vi "IRH1-2M_Heuristic.vi"(10 "Scheduler":T1(ring), 11 "Proocessing Times":u16[][](array[numeric])=[[1, 69, 192, 47, 292, 28, 166, 205], [146, 96, 177, 62, 37, 145, 3, 34], [99, 182, 133, 113, 9, 239, 27, 198], [159, 182, 132, 158, 183, 38, 142, 6], [92, 63, 114, 144, 180, 199, 136, 72], [119, 31, 9, 163, 139, 158, 350, 31], [46, 30, 59, 290, 156, 90, 175, 154], [338, 347, 184, 23, 4, 103, 1, 0]]) -> (3 "IRH1 Schedule":u16[](array[numeric]))   [LabVIEW 2013]
uses:
  Classes/GanntChart.lvclass
panel:
  in  "Proocessing Times (8x8)":u16[][](array[numeric])=[[1, 69, 192, 47, 292, 28, 166, 205], [146, 96, 177, 62, 37, 145, 3, 334], [99, 182, 133, 113, 9, 239, 27, 198], [159, 182, 132, 158, 183, 38, 142, 6], [92, 63, 114, 144, 180, 199, 136, 72], [119, 31, 9, 163, 139, 158, 350, 31], [46, 30, 59, 290, 156, 90, 175, 154], [338, 347, 184, 23, 4, 103, 1, 0]]
  out "Machine Completion Times":u16[](array[numeric])
  out "Completion Times":u16[][](array[numeric])
  out "Job Completion Times":i32[](array[numeric])
  out "String":string
  out "LPT Array":i32[](array[numeric])
  out "Makespan":i32
  # "1, 69, 192, 47, 292, 28, 166, 205], \n[146, 96, 177, 62, 37, 145, 3, 334], \n[99, 182, 133, 113, 9, 239, 27, 198], \n[159, 182, 132, 158, 183, 38, 142, 6], \n[92, 63, 114, 144, 180, 199, 136, 72], \n[119, 31, 9, 163, 139, 158, 350, 31], \n[46, 30, 59, 290, 156, 90, 175, 154], \n[338, 347, 184, 23, 4, 103, 1, 0]]"
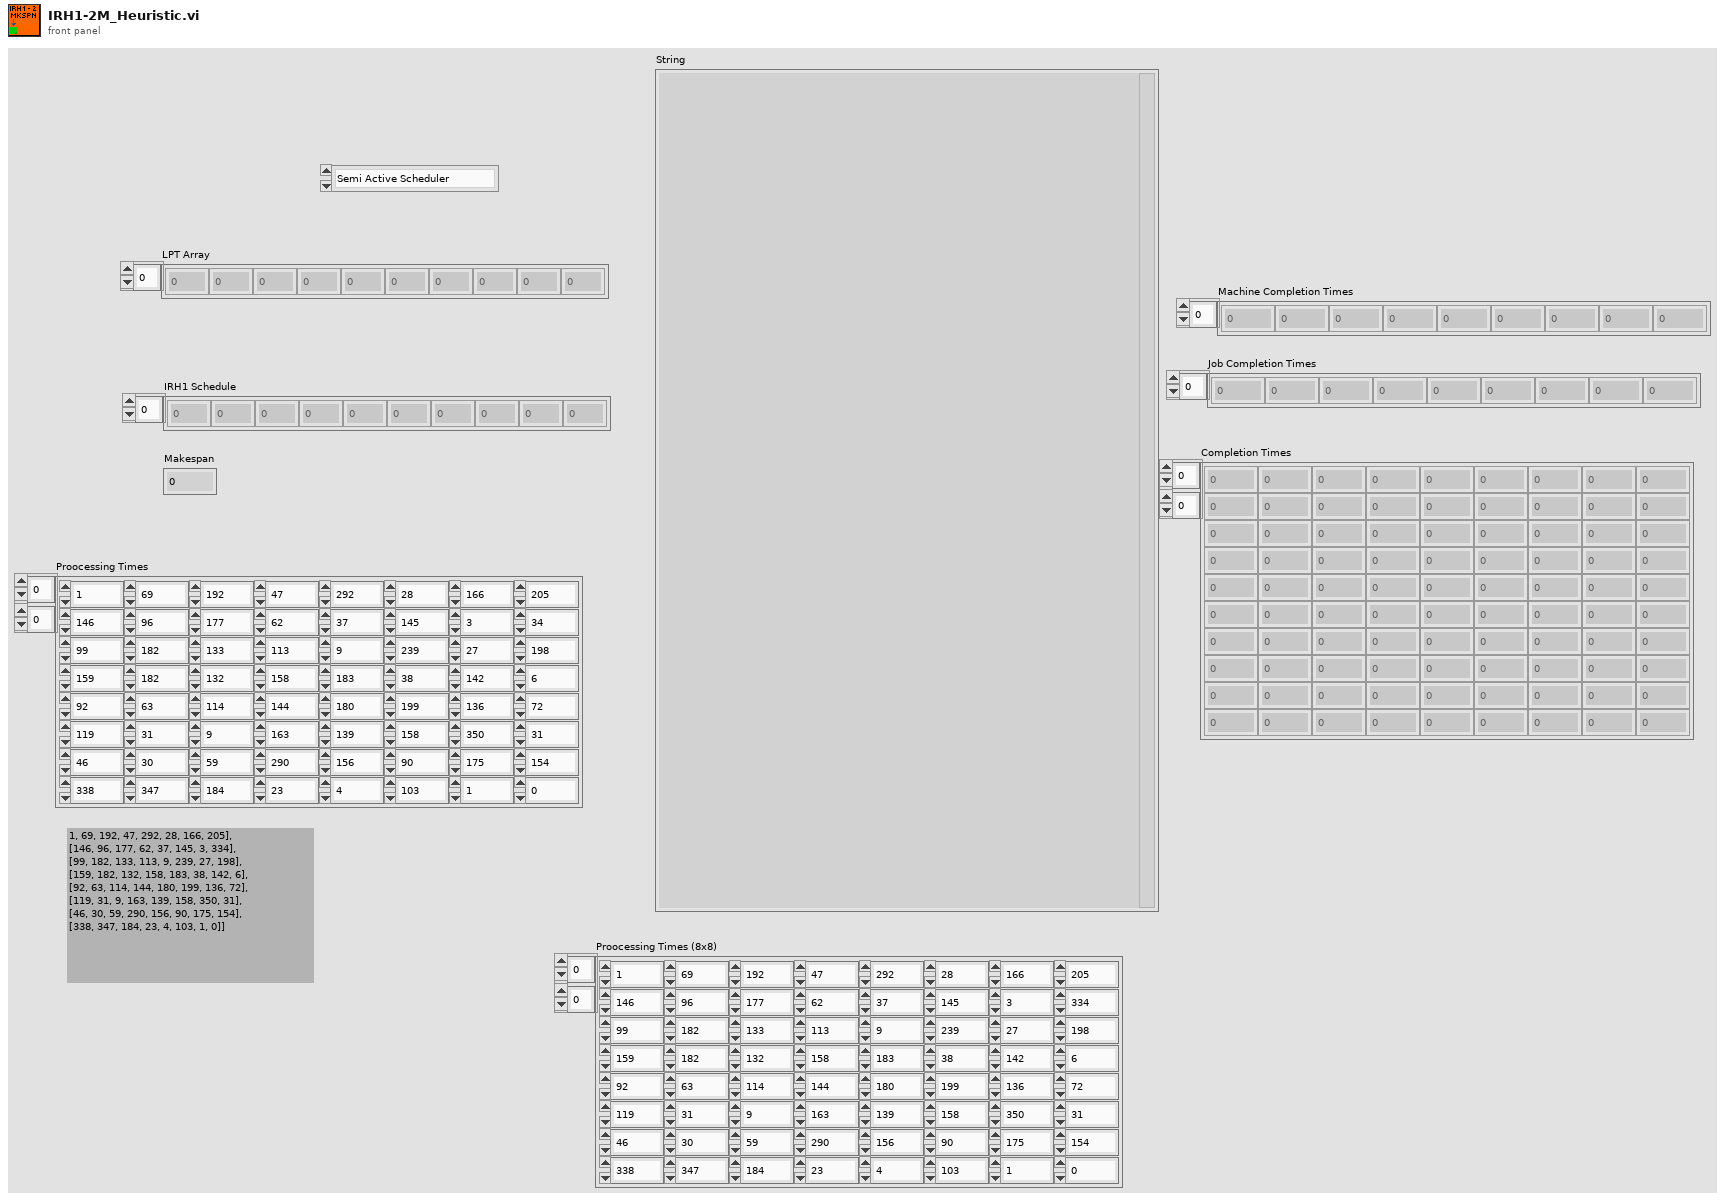
[diagram p1: front panel]
types:
  T1 = enum16{"Semi Active Scheduler", "Non Delay Scheduler"}
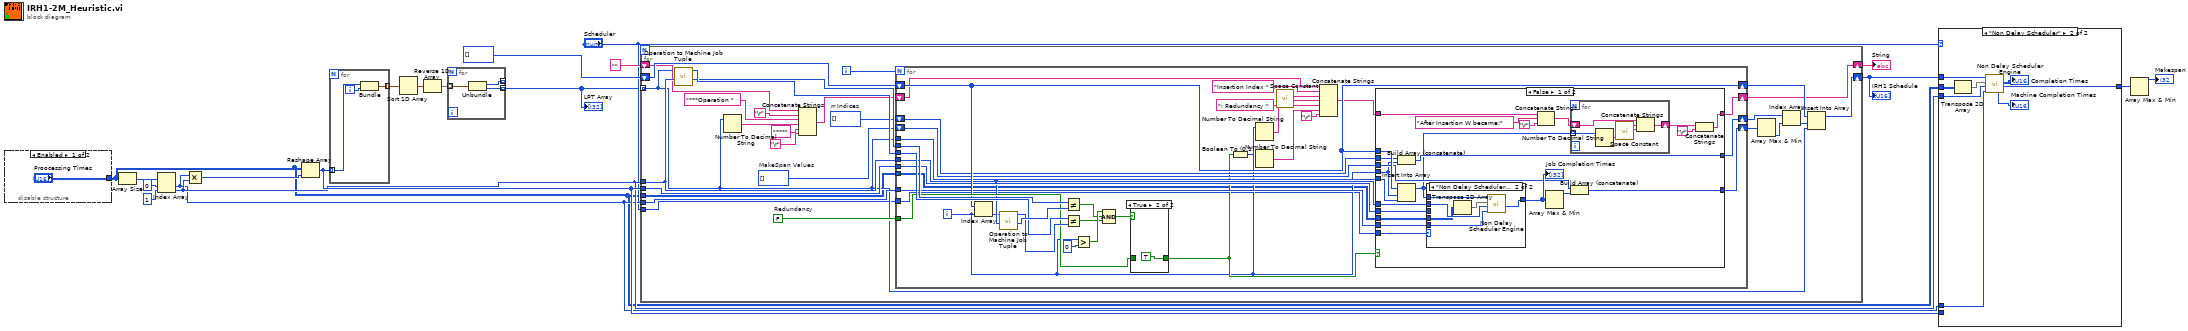
[diagram p0: block diagram]
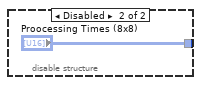
[diagram p2: hidden frame]
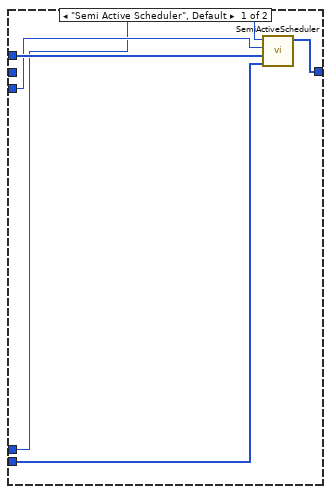
[diagram p3: hidden frame]
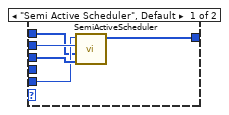
[diagram p4: hidden frame]
diagram:
  n1 = disable-structure shown="Enabled" {
    disable-tunnel: ["Proocessing Times" "Proocessing Times (8x8)"] -> w1
    frame Enabled {
    }
    frame Disabled {
    }
  }
  n2 = Array Size(array=w1) -> (size(s)=w18:i32[])
  n3 = Index Array(array=w18, index #1=0 ("index"), index #2=1 ("index")) -> (element #1=w8:i32, element #2=w9:i32)
  n4 = Multiply(x=w8, y=w9) -> (x*y=w13:i32)
  n5 = Reshape Array(w1, w13) -> (w10:u16[])
  n6 = for {
    tunnel: w10 -> [w24] mode=indexing
    tunnel: [w22] -> w15 mode=indexing
    i -> [w23]
    n7 = Bundle(w24, w23) -> (w22:cluster{u16, i32})  [unwired: 1 in]
  }
  n8 = Sort 1D Array(array=w15) -> (sorted array=w19:cluster{u16, i32}[])
  n9 = Reverse 1D Array(array=w19) -> (reversed array=w14:cluster{u16, i32}[])
  n10 = for {
    tunnel: w14 -> [w27] mode=indexing
    tunnel: [w26] -> _ mode=indexing
    tunnel: [w25] -> w2 mode=indexing
    n11 = Unbundle(w27) -> (w26:u16, w25:i32)
  }
  "LPT Array" <- w2
  n12 = for {
    tunnel: w2 -> [w36] mode=indexing
    tunnel: w9 -> [w48]
    shift-right: [w40] -> w11
    shift-left: u16[] [] -> [w52]
    tunnel: w10 -> [w41]
    tunnel: w8 -> [w47]
    shift-right: [w38] -> w4
    shift-left: "" -> [w37]
    tunnel: w1 -> [w29]
    tunnel: "Scheduler" -> [w28]
    i -> [w54]
    w45 = i32[] []  # MakeSpan Values
    w46 = i32[] []  # rr Indices
    w53 = FALSE  # Redundancy
    n13 = call "Operation to Machine Job Tuple.vi"("Number of Machines"=w48, "Operation Number"=w36) -> ("Job No"=w49:i32, "Machine No"=w50:i32)  [unwired: 8 in]
    n14 = Number To Decimal String(number=w36) -> (decimal integer string=w34:string)  [unwired: 1 in]
    n15 = Concatenate Strings(w37, "\r", "***Operation " ("string"), w34, "***" ("string"), "\r") -> (w33:string)
    n16 = for {
      N: w54 -> [_]
      shift-right: [w79] -> w51
      shift-left: w52 -> [w79]
      tunnel: w50 -> [w83]
      tunnel: w49 -> [w86]
      tunnel: w48 -> [w76]
      tunnel: w53 -> [w80]
      tunnel: w36 -> [w78]
      tunnel: w41 -> [w77]
      tunnel: w47 -> [w75]
      shift-right: [w73] -> w44
      shift-left: w46 -> [w74]
      shift-right: [w71] -> w39
      shift-left: w45 -> [w72]
      shift-right: [w69] -> w38
      shift-left: w33 -> [w63]
      tunnel: w29 -> [w56]
      tunnel: w28 -> [w55]
      i -> [w60]
      n17 = Index Array(array=w79, index=w60) -> (element=w68:u16)
      n18 = call "Operation to Machine Job Tuple.vi"("Number of Machines"=w76, "Operation Number"=w68) -> ("Job No"=w85:i32, "Machine No"=w82:i32)  [unwired: 8 in]
      n19 = Not Equal?(x=w86, y=w85) -> (x != y?=w84:bool)
      n20 = Not Equal?(x=w83, y=w82) -> (x != y?=w70:bool)
      n21 = Greater?(x=w60, y=0) -> (0:w87:bool)
      n22 = Compound Arithmetic op=AND(w87, w84, w70) -> (w81:bool)
      n23 = case shown="True" w81 {
        tunnel: w80 -> [w130 _]
        tunnel: [w130 TRUE ("Redundancy")] -> w61
        frame False {
        }
        frame True {
        }
      }
      n24 = Boolean To (0,1)(Boolean=w61) -> (0, 1=w59:i16)
      n25 = Number To Decimal String(number=w60) -> (decimal integer string=w65:string)  [unwired: 1 in]
      n26 = Number To Decimal String(number=w59) -> (decimal integer string=w58:string)  [unwired: 1 in]
      n27 = call <vilib>:"Space Constant.vi"() -> ("String"=w66:string)
      n28 = Concatenate Strings(w63, "Insertion Index " ("string"), w65, w66, "; Redundancy " ("string"), w58, "\r") -> (w62:string)
      n29 = case shown="False" w61 {
        tunnel: w79 -> [w110 _]
        tunnel: w78 -> [w109 _]
        tunnel: w77 -> [w108 _]
        tunnel: w76 -> [w107 _]
        tunnel: w75 -> [w106 _]
        tunnel: w74 -> [w105 w129]
        tunnel: w60 -> [w97 _]
        tunnel: [w104 w129] -> w73
        tunnel: w72 -> [w102 w128]
        tunnel: [w100 w128] -> w71
        tunnel: [w98 w127] -> w69
        tunnel: w62 -> [w96 w127]
        tunnel: w56 -> [w89 _]
        tunnel: w55 -> [w90 _]
        frame False {
          n30 = Build Array (concatenate)(w105, w97) -> (w104:i32[])
          n31 = Insert Into Array(array=w110, index=w97, new element=w109) -> (w99:u16[])
          n32 = case shown="\"Non Delay Scheduler\"" w90 {
            tunnel: w108 -> [w115 _]
            tunnel: w107 -> [w114 w120]
            tunnel: w106 -> [w113 w119]
            tunnel: [w112 w118] -> w103
            tunnel: w99 -> [w111 w121]
            tunnel: w89 -> [_ w117]
            frame "Semi Active Scheduler", Default {
              n33 = call "SemiActiveScheduler.vi"("Proocessing Times"=w115, "Schedule"=w111, "Number Of Machines"=w114, "Number Of Jobs"=w113) -> ("Job Completion Times"=w112:i32[])  [unwired: 5 in, 2 out]
            }
            frame "Non Delay Scheduler" {
              n34 = Transpose 2D Array(2D array=w117) -> (transposed array=w116:u16[][])
              n35 = call "Non Delay Scheduler Engine.vi"("Number of  Jobs"=w119, "Number of Machines"=w120, "Processing Times"=w116, "Schedule"=w121) -> ("Job Completion Times"=w118:u16[])  [unwired: 3 in, 4 out]
            }
          }
          "Job Completion Times" <- w103
          n36 = Concatenate Strings(w96, "After Insertion W became:" ("string"), "\r") -> (w93:string)
          n37 = Array Max & Min(array=w103) -> (max value=w101:i32)  [unwired: 3 out]
          n38 = for {
            tunnel: w99 -> [w126] mode=indexing
            shift-right: [w123] -> w92
            shift-left: w93 -> [w125]
            n39 = Number To Decimal String(number=w126) -> (decimal integer string=w124:string)  [unwired: 1 in]
            n40 = call <vilib>:"Space Constant.vi"() -> ("String"=w122:string)
            n41 = Concatenate Strings(w125, w124, w122) -> (w123:string)
          }
          n42 = Build Array (concatenate)(w102, w101) -> (w100:i32[])
          n43 = Concatenate Strings(w92, "\r") -> (w98:string)
        }
        frame True {
        }
      }
    }
    n44 = Array Max & Min(array=w39) -> (min index (indices)=w43:i32)  [unwired: 3 out]
    n45 = Index Array(array=w44, index=w43) -> (element=w42:i32)
    n46 = Insert Into Array(array=w51, index=w42, new element=w36) -> (w40:u16[])
  }
  "IRH1 Schedule" <- w11
  "String" <- w4
  n47 = case shown="\"Non Delay Scheduler\"" "Scheduler" {
    tunnel: w11 -> [w136 w144]
    tunnel: w10 -> [w135 _]
    tunnel: w9 -> [w134 w143]
    tunnel: w8 -> [w133 w142]
    tunnel: [w132 w141] -> w7
    tunnel: w1 -> [_ w138]
    frame "Semi Active Scheduler", Default {
      n48 = call "SemiActiveScheduler.vi"("Proocessing Times"=w135, "Schedule"=w136, "Number Of Machines"=w134, "Number Of Jobs"=w133) -> ("Job Completion Times"=w132:i32[])  [unwired: 5 in, 2 out]
    }
    frame "Non Delay Scheduler" {
      n49 = Transpose 2D Array(2D array=w138) -> (transposed array=w137:u16[][])
      n50 = call "Non Delay Scheduler Engine.vi"("Number of  Jobs"=w142, "Number of Machines"=w143, "Processing Times"=w137, "Schedule"=w144) -> ("Job Completion Times"=w141:u16[], "Completion Times"=→"Completion Times":u16[][], "Machine Completion Times"=→"Machine Completion Times":u16[])  [unwired: 3 in, 2 out]
    }
  }
  n51 = Array Max & Min(array=w7) -> (max value=→"Makespan":i32)  [unwired: 3 out]
